vi "MainPICOEnrique.vi"() -> ()   [LabVIEW 2019]
uses:
  PicoData.ctl
  <instrlib>/HandsOnPi2040/Public/AnaIns.ctl
  <instrlib>/HandsOnPi2040/Public/DigIns.ctl
  <instrlib>/HandsOnPi2040/Public/DigOuts.ctl
  <vilib>/PantherLAB/Firebase API/PantherLAB_lib_Filtering Parameters--cluster.ctl
  a087fea8-a487-4c1c-8a8b-15f205e78756.vi
  c90b4970-0cb1-4ed8-a3e8-abf7f56642d0.vi
  079ee137-338a-4224-8d27-3950f07d8dd5.vi
  <vilib>/JDP Science/JSONtext/JSON text to Variant.vi
  <vilib>/JDP Science/JSONtext/LVClass Serializer/JSONtext LVClass Serializer.lvclass
  <vilib>/PantherLAB/Firebase API/PantherLAB_lib_firebase.lvclass
  <vilib>/JDP Science/JSONtext/JSONtext.lvlib
  <instrlib>/HandsOnPi2040/HandsOnPi2040.lvlib
  Shared.lvlib
panel:
  in  "DO":bool[](array[boolean])
  out "DI":bool[](array[boolean])
  in  "Connect":bool
  in  "VISA resource name":refnum<visa-resource-name>="COM3"
  in  "Get All":bool
  in  "Get5":bool
  out "JSON String":string
  in  "Get Newest":bool
  in  "Delete":bool
  in  "Password":string="123456"
  in  "Email":string="enrique.noe@gmail.com"
  in  "Log In":bool
  in  "Sign In":bool
  out "Newest":T1
  out "Data out":T1[](array[typedef])
  out "Pico Analog Signal":u16(graph)
  # "2"
  # "1"
  # "If you are already authenticated\nand you want to start using\nyour Database"
  # "To add an authenticated user\nto your Real Time Database"
  # "Warning:\nThis button will delete all the data\nunder Post EndPoint"
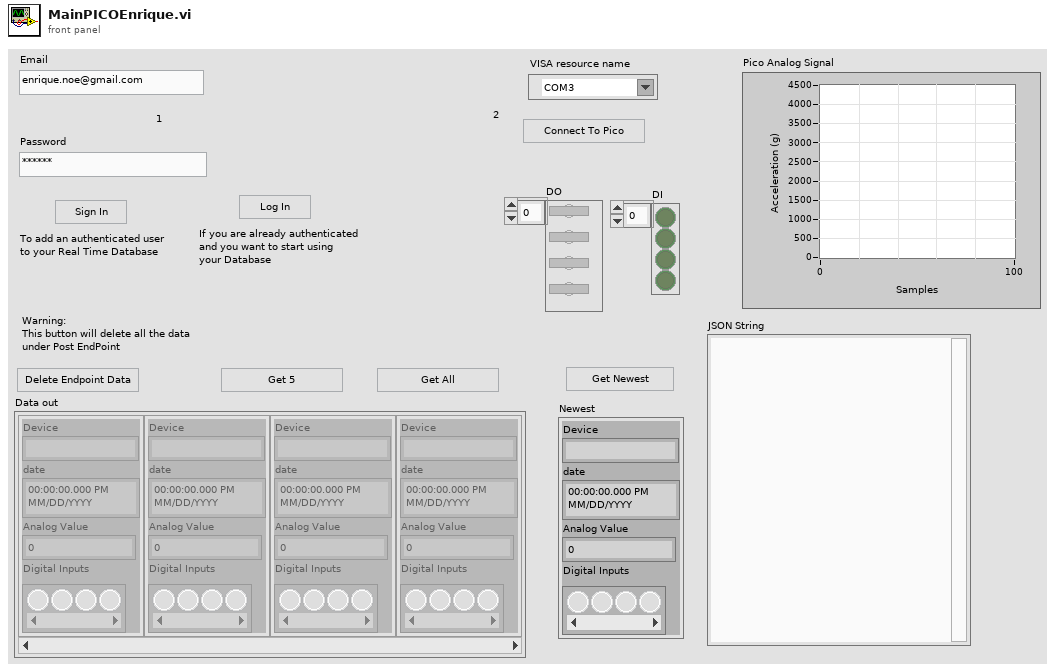
[diagram p1: front panel]
types:
  T1 = typedef "Shared.lvlib/PicoData.ctl" = cluster{"Device":string, "date":timestamp, "Analog Value":u16, "Digital Inputs":bool[]}
  T2 = typedef "HandsOnPi2040.lvlib/AnaIns.ctl" = enum16{"No AI - Error", "AI1 (GPIO26)", "AI2 (GPIO27)"}
  T3 = typedef "PantherLAB_lib_firebase.lvclass/PantherLAB_lib_Filtering Parameters--cluster.ctl" = cluster{"Filtering Param":string, "Argument":string}
  T4 = typedef "HandsOnPi2040.lvlib/DigIns.ctl" = enum16{"No DI - Error", "DI1 (GPIO7)", "DI2 (GPIO8)", "DI3 (GPIO9)", "DI4 (GPIO10)"}
  T5 = typedef "HandsOnPi2040.lvlib/DigOuts.ctl" = enum16{"No DO - Error", "DO1 (GPIO2)", "DO2 (GPIO3)", "DO3 (GPIO4)", "DO4 (GPIO5)", "BEEP (GPIO6)"}
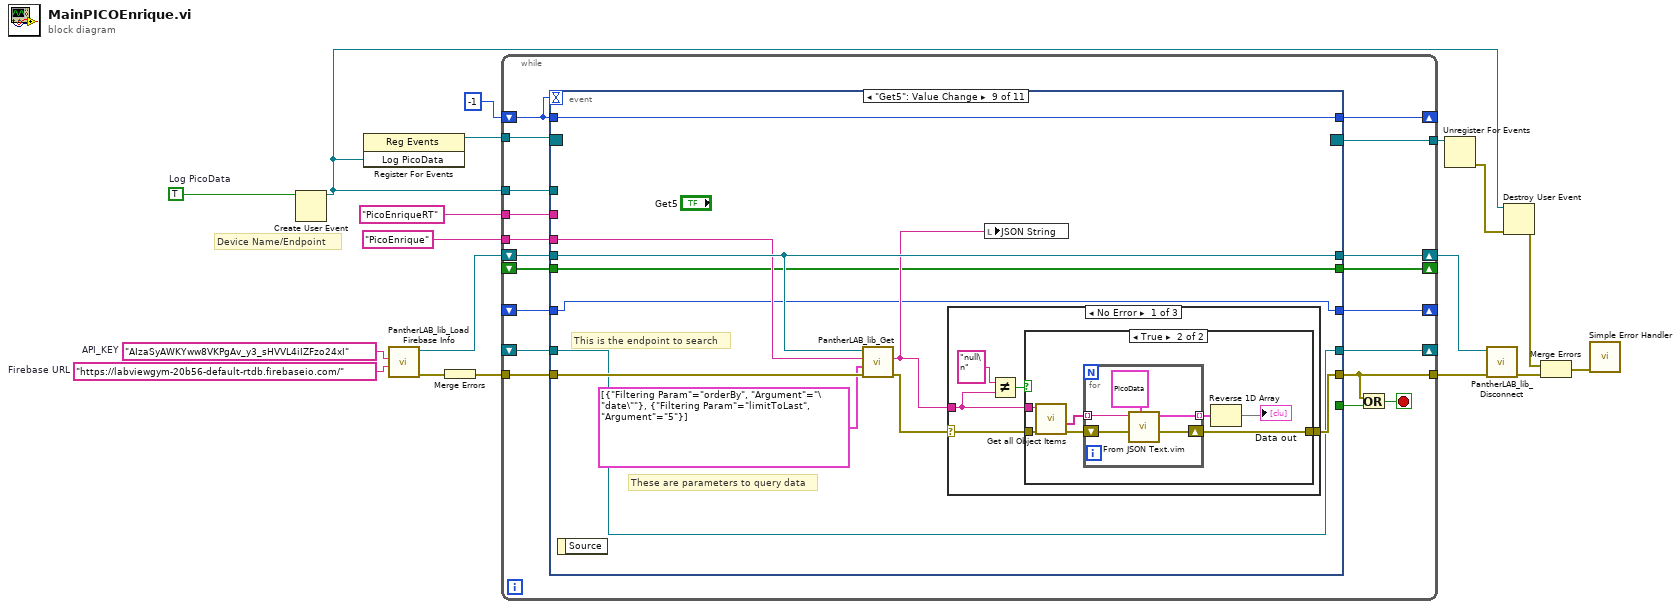
[diagram p0: block diagram]
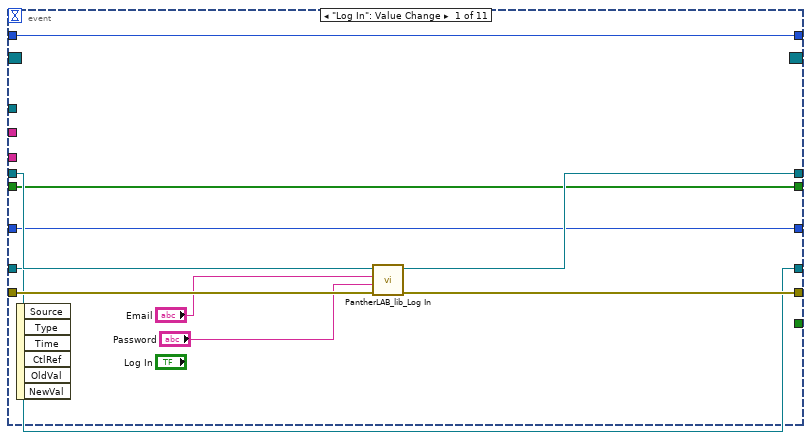
[diagram p2: hidden frame]
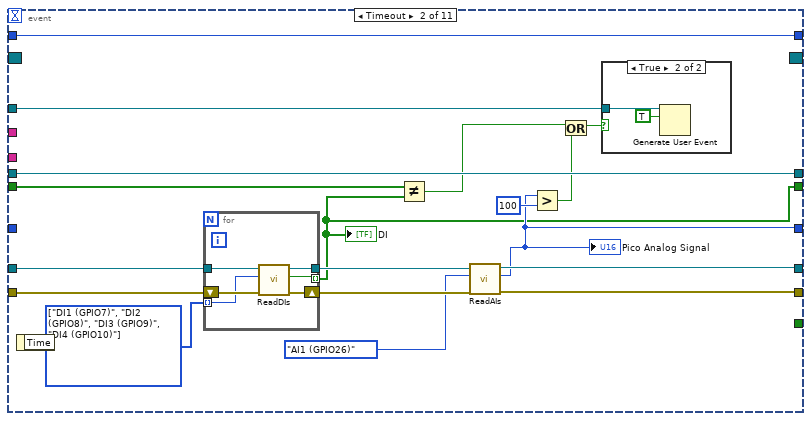
[diagram p3: hidden frame]
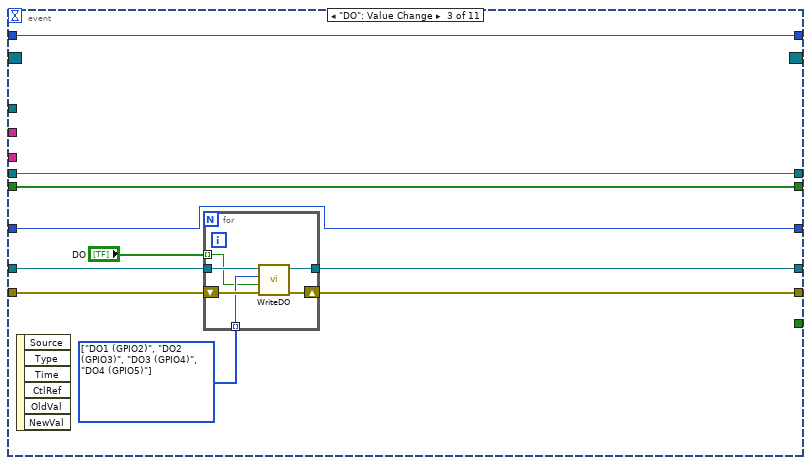
[diagram p5: hidden frame]
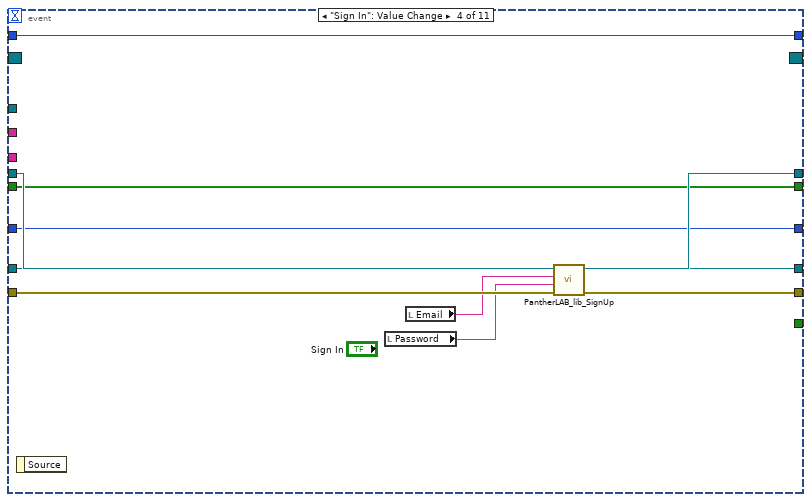
[diagram p6: hidden frame]
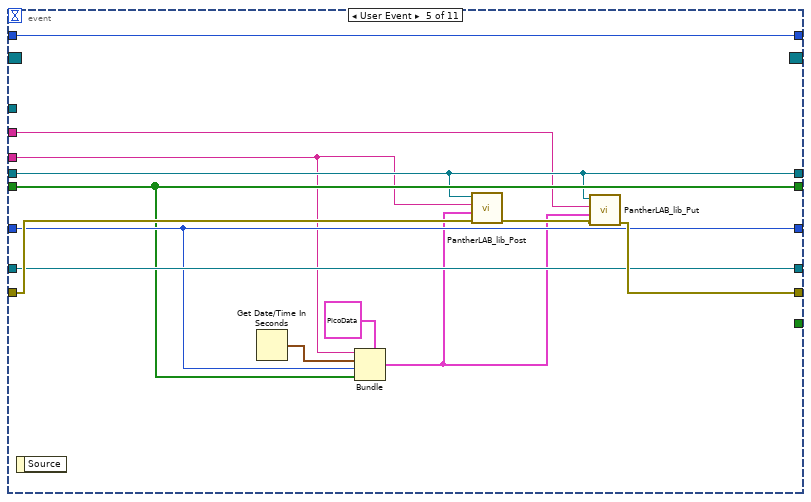
[diagram p7: hidden frame]
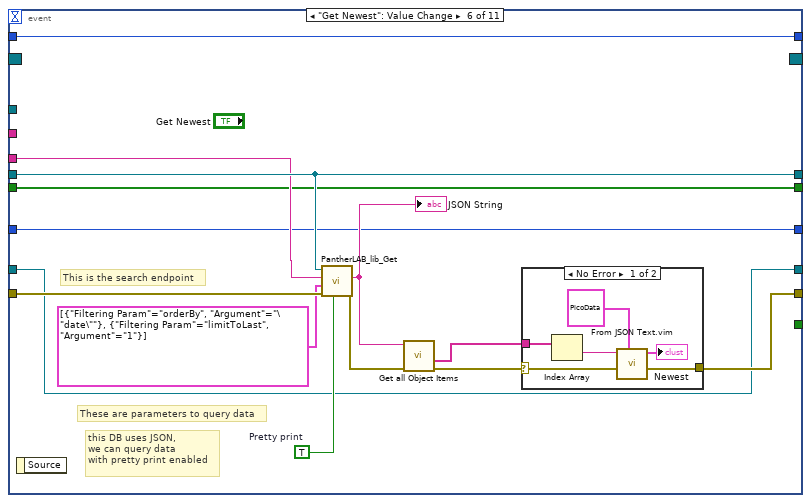
[diagram p8: hidden frame]
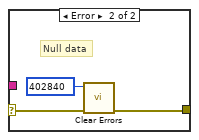
[diagram p9: hidden frame]
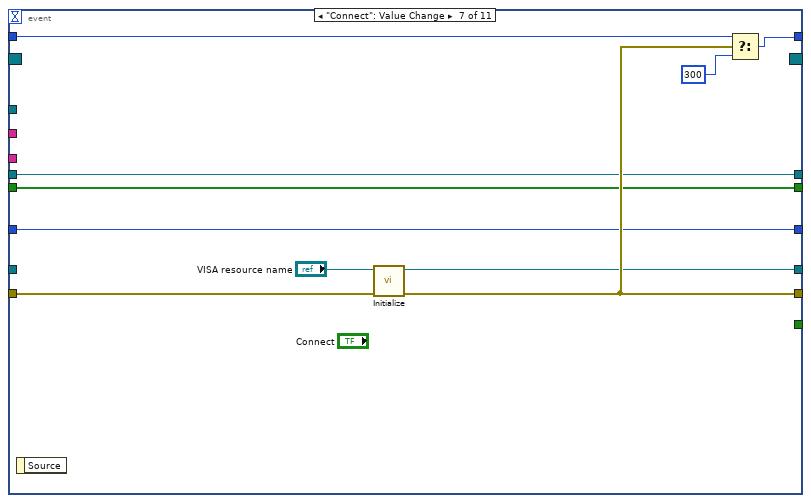
[diagram p10: hidden frame]
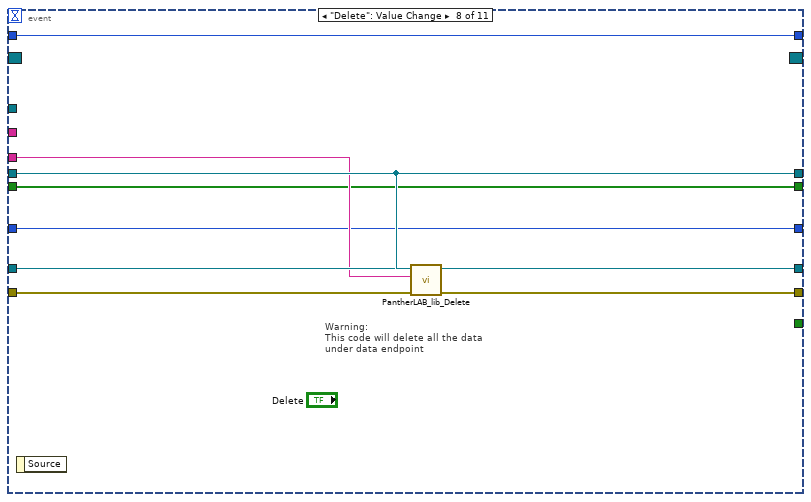
[diagram p11: hidden frame]
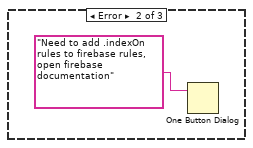
[diagram p13: hidden frame]
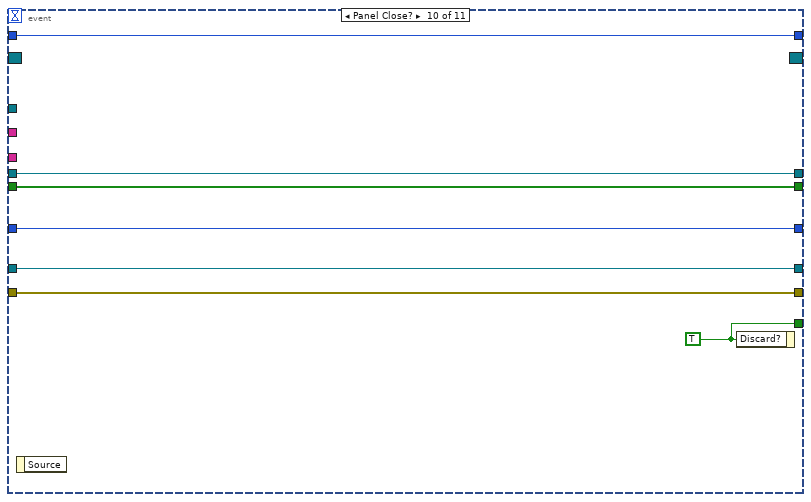
[diagram p15: hidden frame]
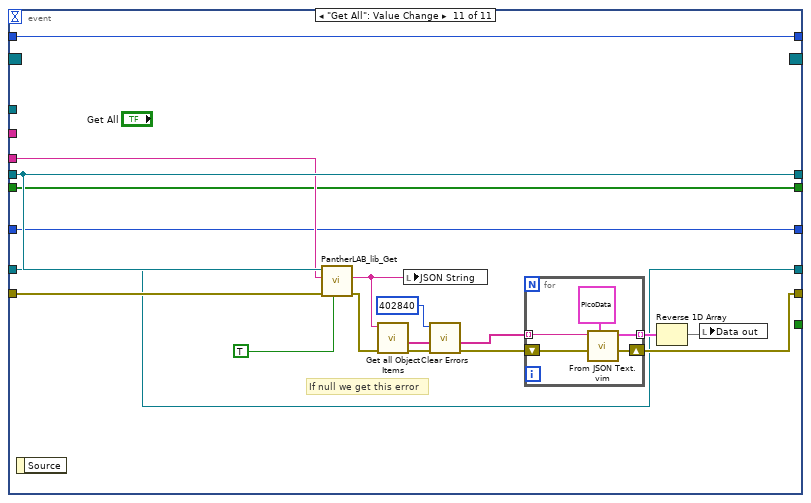
[diagram p16: hidden frame]
diagram:
  w6 = TRUE  # Log PicoData
  w9 = "AIzaSyAWKYww8VKPgAv_y3_sHVVL4iIZFzo24xI"  # API_KEY
  w8 = "https://labviewgym-20b56-default-rtdb.firebaseio.com/"  # Firebase URL
  # "Device Name/Endpoint"
  n1 = Create User Event(user event datatype=w6) -> (user event=w4:refnum<user-event>)  [unwired: 1 in, 1 out]
  n2 = register-events(w4) -> (reference out=w7:refnum<event-registration>)  [unwired: 2 in, 1 out]
  n3 = call <vilib>:"PantherLAB_lib_Load Firebase Info.vi"("Firebase URL"=w8, "API_KEY"=w9) -> ("error out"=w17:errorcluster, "firebase out"=w10:refnum<class "PantherLAB_lib_firebase.lvclass">)  [unwired: 8 in]
  n4 = Merge Errors(w17) -> (w16:errorcluster)
  n5 = while {
    tunnel: w16 -> [w37]
    tunnel: [w36] -> w15
    shift-right: [w32] -> w11
    shift-left: w10 -> [w33]
    shift-right: [w30] -> _
    shift-left: _ -> [w31]
    tunnel: w7 -> [w29]
    tunnel: w4 -> [w28]
    tunnel: [w27] -> w5
    tunnel: "PicoEnrique" -> [w26]
    shift-right: [w25] -> _
    shift-left: _ -> [w24]
    shift-right: [w22] -> _
    shift-left: _ -> [w23]
    shift-right: [w20] -> _
    shift-left: -1 -> [w21]
    tunnel: "PicoEnriqueRT" -> [w19]
    stop <- w34 stop-if-true
    n6 = event shown="[8] \"Get5\": Value Change" {
      selector: w29 -> [_ _ _ _ _ _ _ _ _ _ _]
      dyn-events: [_ _ _ _ _ _ _ _ _ _ _] -> w27
      timeout: w21 -> [_ _ _ _ _ _ _ _ _ _ _]
      tunnel: w37 -> [w47 w64 w83 w99 w112 w126 w145 w153 w164 w191 w208]
      tunnel: [w46 w65 w82 w98 w110 w124 w144 w152 w162 w191 w205] -> w36
      tunnel: [_ _ _ _ _ _ _ _ _ w189 _] -> w35
      tunnel: w33 -> [w43 w62 w81 w95 w103 w119 w143 w151 w160 w190 w198]
      tunnel: [w42 w62 w81 w94 w103 w119 w143 w151 w160 w190 w198] -> w32
      tunnel: w31 -> [w41 w54 w80 w93 w109 w118 _ w150 w159 w188 w197]
      tunnel: [w41 w59 w78 w93 w109 w118 w141 w150 w159 w188 w197] -> w30
      tunnel: w28 -> [_ w61 _ _ _ _ _ _ _ _ _]
      tunnel: w26 -> [_ _ _ _ w102 w117 _ w149 w158 _ w196]
      tunnel: [w40 w56 w77 w92 w107 w115 w140 w148 w156 w187 w194] -> w25
      tunnel: w24 -> [w40 _ w77 w92 w107 w115 w140 w148 w156 w187 w194]
      tunnel: w23 -> [w39 w50 w74 w91 w106 w114 w139 w147 w155 w186 w193]
      tunnel: [w39 w49 w74 w91 w106 w114 w139 w147 w155 w186 w193] -> w22
      tunnel: w21 -> [w38 w48 w79 w90 w104 w113 w138 w146 w154 w185 w192]
      tunnel: [w38 w48 w79 w90 w104 w113 w137 w146 w154 w185 w192] -> w20
      tunnel: w19 -> [_ _ _ _ w100 _ _ _ _ _ _]
      event "Log In": Value Change {
        n7 = event-data() -> ()  [unwired: 1 in, 6 out]
        n8 = call-dynamic "PantherLAB_lib_Log In.vi"("error in"=w47, "password"="Password", "email"="Email", "firebase in"=w43) -> ("error out"=w46:errorcluster, "firebase out"=w42:refnum<class "PantherLAB_lib_firebase.lvclass">)  [unwired: 6 in]
      }
      event Timeout {
        w55 = T4[] [enum."DI1 (GPIO7)", enum."DI2 (GPIO8)", enum."DI3 (GPIO9)", enum."DI4 (GPIO10)"] items=["No DI - Error", "DI1 (GPIO7)", "DI2 (GPIO8)", "DI3 (GPIO9)", "DI4 (GPIO10)"] ("Array")
        n9 = event-data() -> ()  [unwired: 1 in, 1 out]
        n10 = for {
          tunnel: w55 -> [w69] mode=indexing
          tunnel: w54 -> [w68]
          tunnel: [w67] -> w53
          shift-right: [w70] -> w63
          shift-left: w64 -> [w71]
          tunnel: [w66] -> w49 mode=indexing
          n11 = call <instrlib>:"ReadDIs.vi"("error in (no error)"=w71, "Digital Inputs"=w69, "VISA resource name"=w68) -> ("error out"=w70:errorcluster, "DIStatus"=w66:bool, "VISA resource name out"=w67:refnum<visa-resource-name>)  [unwired: 6 in]
        }
        "DI" <- w49
        n12 = Not Equal?(x=w50, y=w49) -> (x != y?=w51:bool)
        n13 = call <instrlib>:"ReadAIs.vi"("error in (no error)"=w63, "Analog Inputs"=AnaIns."AI1 (GPIO26)", "VISA resource name"=w53) -> ("error out"=w65:errorcluster, "Value"=w56:u16, "VISA resource name out"=w59:refnum<visa-resource-name>)  [unwired: 6 in]
        "Pico Analog Signal" <- w56
        n14 = Greater?(x=w56, y=u16 100) -> (0:w57:bool)
        n15 = Or(x=w51, y=w57) -> (x .or. y?=w52:bool)
        n16 = case shown="True" w52 {
          tunnel: w61 -> [_ w73]
          frame False {
          }
          frame True {
            n17 = Generate User Event(user event=w73, event data cluster=TRUE ("event data")) -> ()  [unwired: 2 in, 2 out]
          }
        }
      }
      event "DO": Value Change {
        w76 = T5[] [enum."DO1 (GPIO2)", enum."DO2 (GPIO3)", enum."DO3 (GPIO4)", enum."DO4 (GPIO5)"] items=["No DO - Error", "DO1 (GPIO2)", "DO2 (GPIO3)", "DO3 (GPIO4)", "DO4 (GPIO5)", "BEEP (GPIO6)"] ("Array")
        n18 = event-data() -> ()  [unwired: 1 in, 6 out]
        n19 = for {
          tunnel: w80 -> [w87]
          tunnel: [w86] -> w78
          shift-right: [w88] -> w82
          shift-left: w83 -> [w89]
          tunnel: w76 -> [w85] mode=indexing
          tunnel: "DO" -> [w84] mode=indexing
          n20 = call <instrlib>:"WriteDO.vi"("error in (no error)"=w89, "DO Value (True)"=w84, "Output"=w85, "VISA resource name"=w87) -> ("error out"=w88:errorcluster, "VISA resource name out"=w86:refnum<visa-resource-name>)  [unwired: 6 in]
        }
      }
      event "Sign In": Value Change {
        n21 = event-data() -> ()  [unwired: 1 in, 1 out]
        n22 = local read "Password"() -> (w97:string)
        n23 = local read "Email"() -> (w96:string)
        n24 = call-dynamic "PantherLAB_lib_SignUp.vi"("error in"=w99, "password"=w97, "email"=w96, "firebase in"=w95) -> ("error out"=w98:errorcluster, "firebase out"=w94:refnum<class "PantherLAB_lib_firebase.lvclass">)  [unwired: 6 in]
      }
      event User Event {
        n25 = event-data() -> ()  [unwired: 1 in, 1 out]
        n26 = Get Date/Time In Seconds() -> (seconds since 1Jan1904=w108:timestamp)
        n27 = Bundle(cluster=T1 {"Device"="", "date"=timestamp(0 s since 1904-01-01), "Analog Value"=0, "Digital Inputs"=[]} ("output cluster"), "Device"=w102, "date"=w108, "Analog Value"=w107, "Digital Inputs"=w106) -> (w101:T1)
        n28 = call-dynamic "PantherLAB_lib_Post.vi"("error in"=w112, "Anything"=w101, "endPoint"=w102, "firebase in"=w103) -> ("error out"=w111:errorcluster)  [unwired: 6 in, 1 out]
        n29 = call-dynamic "PantherLAB_lib_Put.vi"("error in"=w111, "Anything"=w101, "endPoint"=w100, "firebase in"=w103) -> ("error out"=w110:errorcluster)  [unwired: 6 in, 1 out]
      }
      event "Get Newest": Value Change {
        w120 = TRUE  # Pretty print
        # "this DB uses JSON,\nwe can query data\nwith pretty print enabled"
        # "These are parameters to query data"
        # "This is the search endpoint"
        n30 = event-data() -> ()  [unwired: 1 in, 1 out]
        n31 = call-dynamic "PantherLAB_lib_Get.vi"("Pretty print"=w120, "error in"=w126, "Filtering Params"=T3[] [{"Filtering Param"="orderBy", "Argument"="\"date\""}, {"Filtering Param"="limitToLast", "Argument"="1"}], "endPoint"=w117, "firebase in"=w119) -> ("error out"=w125:errorcluster, "Json String"=w121:string)  [unwired: 5 in]
        "JSON String" <- w121
        n32 = call <vilib>:"Get all Object Items.vi"("error in (no error)"=w125, "JSON"=w121) -> ("error out"=w123:errorcluster, "<JSON>"=w116:string[])  [unwired: 6 in, 2 out]
        n33 = case shown="No Error" w123 {
          selector: w123 -> [w132 w135]
          tunnel: [w131 w134] -> w124
          tunnel: w116 -> [w130 _]
          frame No Error {
            n34 = Index Array(array=w130) -> (element=w129:string)  [unwired: 1 in]
            n35 = call "From JSON Text.vim"("Data Type and Default Value"=T1 {"Device"="", "date"=timestamp(0 s since 1904-01-01), "Analog Value"=0, "Digital Inputs"=[]} ("output cluster"), "error in (no error)"=w132, "JSON"=w129) -> ("error out"=w131:errorcluster, "Data out"=→"Newest":T1)  [unwired: 7 in]
          }
          frame Error {
            # "Null data"
            n36 = call <vilib>:"Clear Errors.vi"("error in (no error)"=w135, "specific error code to clear (0: all)"=402840) -> ("error out"=w134:errorcluster)  [unwired: 4 in, 1 out]
          }
        }
      }
      event "Connect": Value Change {
        n37 = event-data() -> ()  [unwired: 1 in, 1 out]
        n38 = call <instrlib>:"Initialize.vi"("error in (no error)"=w145, "VISA resource name"="VISA resource name") -> ("error out"=w144:errorcluster, "VISA resource name out"=w141:refnum<visa-resource-name>)  [unwired: 7 in, 1 out]
        n39 = Select(t=w138, s=w144, f=300) -> (s? t:f=w137:i32)
      }
      event "Delete": Value Change {
        # "Warning:\nThis code will delete all the data\nunder data endpoint"
        n40 = event-data() -> ()  [unwired: 1 in, 1 out]
        n41 = call-dynamic "PantherLAB_lib_Delete.vi"("error in"=w153, "endPoint"=w149, "firebase in"=w151) -> ("error out"=w152:errorcluster)  [unwired: 7 in, 1 out]
      }
      event "Get5": Value Change {
        # "This is the endpoint to search"
        # "These are parameters to query data"
        n42 = event-data() -> ()  [unwired: 1 in, 1 out]
        n43 = call-dynamic "PantherLAB_lib_Get.vi"("error in"=w164, "Filtering Params"=T3[] [{"Filtering Param"="orderBy", "Argument"="\"date\""}, {"Filtering Param"="limitToLast", "Argument"="5"}], "endPoint"=w158, "firebase in"=w160) -> ("error out"=w163:errorcluster, "Json String"=w157:string)  [unwired: 6 in]
        n44 = case shown="No Error" w163 {
          selector: w163 -> [w169 _ w184]
          tunnel: [w168 _ w184] -> w162
          tunnel: w157 -> [w165 _ _]
          frame No Error {
            n45 = Not Equal?(x="null\n" ("Display"), y=w165) -> (x != y?=w166:bool)
            n46 = case shown="True" w166 {
              tunnel: w169 -> [w170 w176]
              tunnel: [w170 w175] -> w168
              tunnel: w165 -> [_ w172]
              frame False {
                # "No data"
              }
              frame True {
                n47 = call <vilib>:"Get all Object Items.vi"("error in (no error)"=w176, "JSON"=w172) -> ("error out"=w177:errorcluster, "<JSON>"=w174:string[])  [unwired: 6 in, 2 out]
                n48 = for {
                  tunnel: w174 -> [w180] mode=indexing
                  shift-right: [w181] -> w175
                  shift-left: w177 -> [w182]
                  tunnel: [w179] -> w173 mode=indexing
                  n49 = call "From JSON Text.vim"("Data Type and Default Value"=T1 {"Device"="", "date"=timestamp(0 s since 1904-01-01), "Analog Value"=0, "Digital Inputs"=[]} ("Pico Data"), "error in (no error)"=w182, "JSON"=w180) -> ("error out"=w181:errorcluster, "Data out"=w179:T1)  [unwired: 7 in]
                }
                n50 = Reverse 1D Array(array=w173) -> (reversed array=→"Data out":T1[])
              }
            }
          }
          frame Error {
            n51 = One Button Dialog(message="Need to add .indexOn rules to firebase rules, open firebase documentation") -> ()  [unwired: 1 in, 1 out]
          }
          frame Default {
          }
        }
        n52 = local write "JSON String"(w157) -> ()
      }
      event Panel Close? {
        w189 = TRUE ("Discard?")
        n53 = event-data() -> ()  [unwired: 1 in, 1 out]
        n54 = event-data("Discard?"=w189) -> ()  [unwired: 1 in, 1 out]
      }
      event "Get All": Value Change {
        # "If null we get this error"
        n55 = event-data() -> ()  [unwired: 1 in, 1 out]
        n56 = call-dynamic "PantherLAB_lib_Get.vi"("Pretty print"=TRUE, "error in"=w208, "endPoint"=w196, "firebase in"=w198) -> ("error out"=w206:errorcluster, "Json String"=w201:string)  [unwired: 6 in]
        n57 = call <vilib>:"Get all Object Items.vi"("error in (no error)"=w206, "JSON"=w201) -> ("error out"=w207:errorcluster, "<JSON>"=w203:string[])  [unwired: 6 in, 2 out]
        n58 = local write "JSON String"(w201) -> ()
        n59 = call <vilib>:"Clear Errors.vi"("error in (no error)"=w207, "specific error code to clear (0: all)"=402840) -> ("error out"=w204:errorcluster)  [unwired: 4 in, 1 out]
        n60 = for {
          tunnel: w203 -> [w211] mode=indexing
          shift-right: [w212] -> w205
          shift-left: w204 -> [w213]
          tunnel: [w210] -> w202 mode=indexing
          n61 = call "From JSON Text.vim"("Data Type and Default Value"=T1 {"Device"="", "date"=timestamp(0 s since 1904-01-01), "Analog Value"=0, "Digital Inputs"=[]} ("Pico Data"), "error in (no error)"=w213, "JSON"=w211) -> ("error out"=w212:errorcluster, "Data out"=w210:T1)  [unwired: 7 in]
        }
        n62 = Reverse 1D Array(array=w202) -> (reversed array=w195:T1[])
        n63 = local write "Data out"(w195) -> ()
      }
    }
    n64 = Or(x=w36, y=w35) -> (x .or. y?=w34:bool)
  }
  n65 = Unregister For Events(event registration refnum=w5) -> (error out=w12:errorcluster)  [unwired: 1 in]
  n66 = call-dynamic "PantherLAB_lib_Disconnect.vi"("error in"=w15, "firebase in"=w11) -> ("error out"=w18:errorcluster)  [unwired: 9 in]
  n67 = Destroy User Event(user event=w4, error in=w12) -> (error out=w13:errorcluster)
  n68 = Merge Errors(w13, w18) -> (w14:errorcluster)
  n69 = call <vilib>:"Simple Error Handler.vi"("error in (no error)"=w14) -> ()  [unwired: 4 in, 5 out]
